vi "Bookmarks.vi"(8 "error in (no error)":errorcluster, 11 "NI_report in":refnum<class "NI_report.lvclass">) -> (0 "error out":errorcluster, 2 "Array":string[](array[string]), 3 "NI_report out":refnum<class "NI_report.lvclass">)   [LabVIEW 2018, in "WordReportGeneration.lvlib" / "Word_Report.lvclass"]
uses:
  Word_Report.lvclass
  <vilib>/Utility/NIReport.llb/NI_report.lvclass
  <vilib>/Utility/NIReport.llb/Word/NI_Word.lvclass
  WordReportGeneration.lvlib
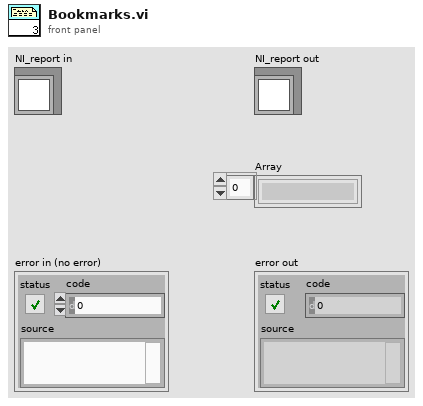
[diagram p1: front panel]
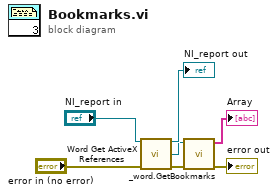
[diagram p0: block diagram]
diagram:
  n1 = call <vilib>:"Word Get ActiveX References.vi"("report in"="NI_report in", "error in (no error)"="error in (no error)") -> ("report out"=→"NI_report out":refnum<class "NI_report.lvclass">, "Word._Document"=w3:refnum<k7>, "error out"=w4:errorcluster)  [unwired: 7 in, 4 out]
  n2 = call "_word.GetBookmarks.vi"("error in (no error)"=w4, "Automation Refnum in"=w3) -> ("error out"=→"error out":errorcluster, "Array"=→"Array":string[])  [unwired: 8 in]
